vi "Limit Remote Front Panel Connections (NI Example).vi"() -> ()   [LabVIEW 2024]
panel:
  in  "Limit Client connections":i32=1 min=1
  in  "stop":bool
  out "Numeric":dbl
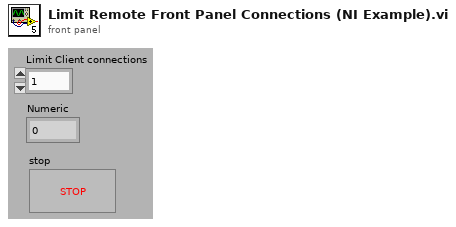
[diagram p1: front panel]
types:
  T1 = typedef "LVRemotePanelConnectionsTypeDef.ctl" = cluster{"VI Name":string, "Remote":string, "UserName":string, "Port":i32, "Status":enum32{"Viewing", "Waiting For Control", "Controlling"}, "Create Time":timestamp, "Status Time":timestamp, "Control End Time":timestamp}[]
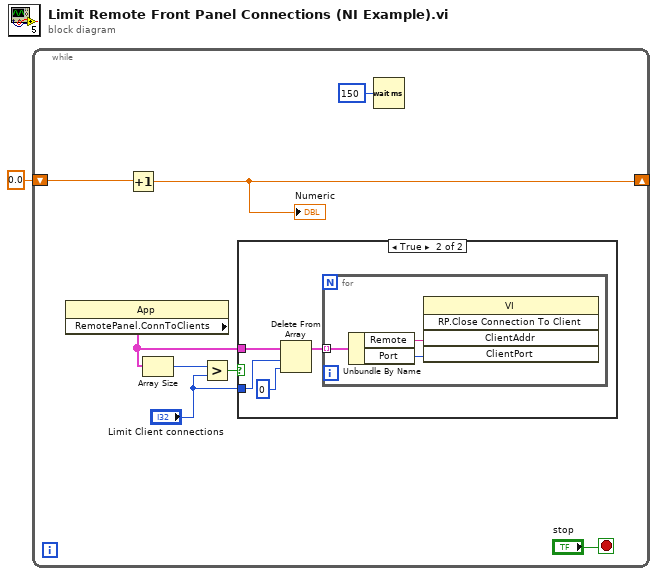
[diagram p0: block diagram]
diagram:
  n1 = while {
    shift-right: [w3] -> _
    shift-left: 0.0 -> [w4]
    stop <- "stop" stop-if-true
    n2 = property class="App"() -> ("RemotePanel.ConnToClients"=w7:T1)  [unwired: 2 in, 2 out]
    n3 = Increment(x=w4) -> (x+1=w3:dbl)
    "Numeric" <- w3
    n4 = Array Size(array=w7) -> (size(s)=w9:i32)
    n5 = Greater?(x=w9, y="Limit Client connections") -> (0:w8:bool)
    n6 = case shown="True" w8 {
      tunnel: w7 -> [_ w13]
      tunnel: "Limit Client connections" -> [_ w10]
      frame False {
      }
      frame True {
        n7 = Delete From Array(array=w13, length=w10, index=0) -> (array with subset deleted=w11:T1)  [unwired: 1 out]
        n8 = for {
          tunnel: w11 -> [w16] mode=indexing
          n9 = Unbundle By Name(w16) -> ("Remote"=w15:string, "Port"=w14:i32)
          n10 = invoke class="VI" method="RP.Close Connection To Client"("ClientAddr"=w15, "ClientPort"=w14) -> ()  [unwired: 3 in, 5 out]
        }
      }
    }
    n11 = Wait (ms)(milliseconds to wait=u32 150) -> ()  [unwired: 1 out]
  }
